vi "TCP Msg Server.vi"() -> ()   [LabVIEW 2020]
uses:
  <vilib>/IlluminatedG/lv-stream-tcp/TCP Server/TCP Server.lvclass
  C:/Program Files (x86)/National Instruments/LabVIEW 2020/vi.lib/IlluminatedG/lv-stream/Endpoint/Endpoint.lvclass
  bda473c8-1423-4ab2-b01a-ba1dcfa4ad6d.vi
  f62ccf13-e430-49b0-9820-5d38b530824a.vi
  bda473c8-1423-4ab2-b01a-ba1dcfa4ad6d.vi/43e93f4b-eb60-4448-b7e4-56a49cc750fb.vi
  f62ccf13-e430-49b0-9820-5d38b530824a.vi/43e93f4b-eb60-4448-b7e4-56a49cc750fb.vi
  bda473c8-1423-4ab2-b01a-ba1dcfa4ad6d.vi/43e93f4b-eb60-4448-b7e4-56a49cc750fb.vi/4b61994f-5270-44fc-a580-5e93e6c23fba.vi
  f62ccf13-e430-49b0-9820-5d38b530824a.vi/43e93f4b-eb60-4448-b7e4-56a49cc750fb.vi/4b61994f-5270-44fc-a580-5e93e6c23fba.vi
  <vilib>/IlluminatedG/lv-stream/stream/Write Formatted Data.vi
  <vilib>/IlluminatedG/lv-msg-simple/Stream-Simple-Msg/Manager/Get Endpoints.vi
  <vilib>/IlluminatedG/lv-msg-simple/Stream-Simple-Msg/Endpoint/Get Stream.vi
  <vilib>/IlluminatedG/lv-stream/stream/Get Mode.vi
  <vilib>/IlluminatedG/lv-stream/stream/Prepared.vi
  <vilib>/Utility/error.llb/Error Cluster From Error Code.vi
  <vilib>/IlluminatedG/lv-stream/stream/Dispatch Sniffer Data.vi
  <vilib>/IlluminatedG/lv-stream/stream/Stream.lvclass
  <vilib>/IlluminatedG/lv-stream/Endpoint/Endpoint.lvclass
  <vilib>/IlluminatedG/lv-msg-simple/Stream-Simple-Msg/Manager/Manager.lvclass
panel:
  out "Connected":bool
  out "error out":errorcluster
  in  "Slide":dbl(slide) scale=0.0..10.0
  in  "Stop":bool
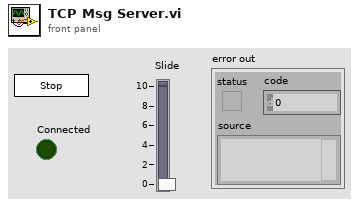
[diagram p1: front panel]
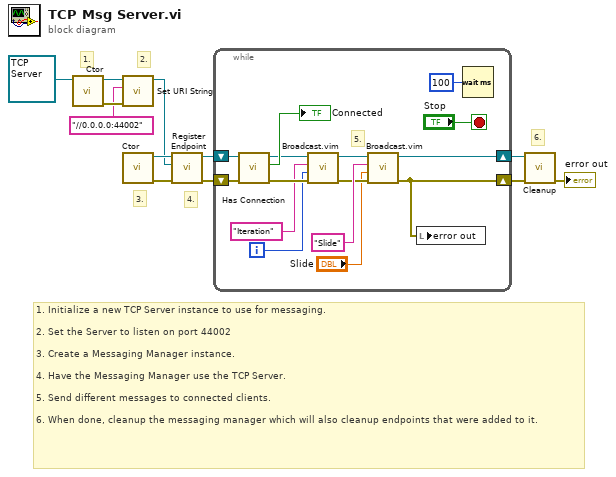
[diagram p0: block diagram]
diagram:
  # "6."
  # "1. Initialize a new TCP Server instance to use for messaging.\n\n2. Set the Server to listen on port 44002\n\n3. Create a Messaging Manager instance.\n\n4. Have the Messaging Manager use the TCP Server.\n\n5. Send different messages to connected clients.\n\n6. When done, cleanup the messaging manager which will also cleanup endpoints that were added to it."
  # "4."
  # "3."
  # "2."
  # "1."
  n1 = call-dynamic <vilib>:"Ctor.vi"("TCP Server in"=refnum<class "TCP Server.lvclass"> refnum) -> ("error out"=w9:errorcluster, "TCP Server out"=w10:refnum<class "TCP Server.lvclass">)  [unwired: 9 in]
  n2 = call <vilib>:"Set URI String.vi"("error in (no error)"=w9, "URI String"="//0.0.0.0:44002", "Endpoint in"=w10) -> ("Endpoint out"=w1:refnum<class "TCP Server.lvclass">)  [unwired: 7 in, 1 out]
  n3 = call <vilib>:"Ctor.vi"() -> ("error out"=w4:errorcluster, "Manager out"=w7:refnum<class "Manager.lvclass">)  [unwired: 10 in]
  n4 = call <vilib>:"Register Endpoint.vi"("error in (no error)"=w4, "Stream:Endpoint"=w1, "Manager in"=w7) -> ("error out"=w12:errorcluster, "Manager out"=w6:refnum<class "Manager.lvclass">)  [unwired: 7 in]
  n5 = while {
    shift-right: [w26] -> w5
    shift-left: w6 -> [w23]
    shift-right: [w24] -> w3
    shift-left: w12 -> [w22]
    i -> [w14]
    stop <- "Stop" stop-if-true
    # "5."
    n6 = call <vilib>:"Has Connection.vi"("error in (no error)"=w22, "Manager in"=w23) -> ("error out"=w18:errorcluster, "Connected"=→"Connected":bool, "Manager out"=w19:refnum<class "Manager.lvclass">)  [unwired: 7 in]
    n7 = call "Broadcast.vim"("error in (no error)"=w18, "Data"=w14, "ID"="Iteration", "Manager in"=w19) -> ("error out"=w17:errorcluster, "Manager out"=w16:refnum<class "Manager.lvclass">)  [unwired: 6 in]
    n8 = call "Broadcast.vim"("error in (no error)"=w17, "Data"="Slide", "ID"="Slide", "Manager in"=w16) -> ("error out"=w24:errorcluster, "Manager out"=w26:refnum<class "Manager.lvclass">)  [unwired: 6 in]
    n9 = local write "error out"(w24) -> ()
    n10 = Wait (ms)(milliseconds to wait=u32 100) -> ()  [unwired: 1 out]
  }
  n11 = call <vilib>:"Cleanup.vi"("error in (no error)"=w3, "Manager in"=w5) -> ("error out"=→"error out":errorcluster)  [unwired: 9 in]
